vi "TDMS_CalcSize.vi"(7 "游标设定":T1={"初始Offset"=0, "每隔多少点读一次"=100000, "每次读的点数"=128}, 8 "错误输入":errorcluster, 9 "Cur2":cluster{"X":dbl, "Y":dbl}={"X"=31490.774276845874, "Y"=-0.08000000000000003}, 10 "Cur1":cluster{"X":dbl, "Y":dbl}={"X"=55721.10494959388, "Y"=0.43999999999999984}, 11 "tdms文件":refnum<k34>) -> (0 "错误输出":errorcluster, 1 "大于300M":bool, 2 "数据大小(MB)":dbl=1.7309100138019612e+18, 3 "tdms out":refnum<k34>)   [LabVIEW 2011]
panel:
  in  "通道名":string[](array[string])=["Sinc", "Sin"]
  in  "组名称输入":string="Sig Group"
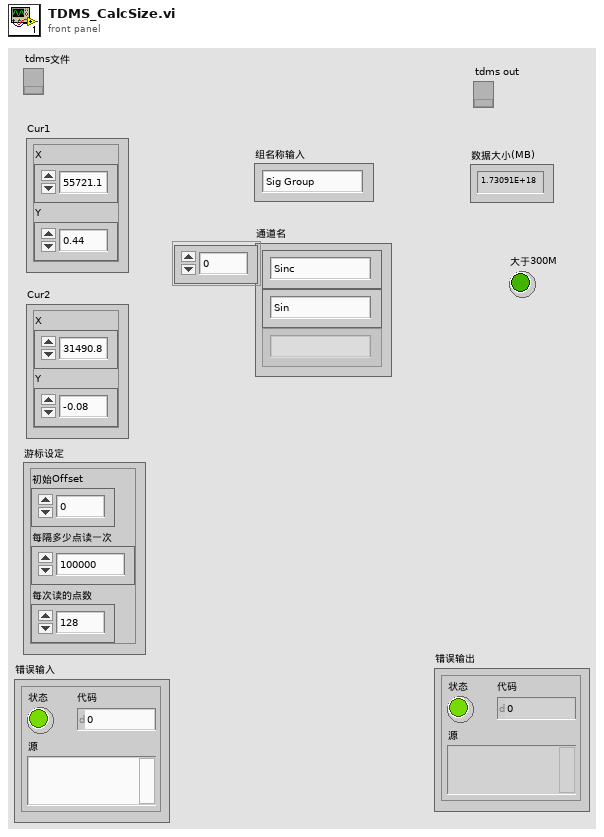
[diagram p1: front panel]
types:
  T1 = cluster{"初始Offset":u64, "每隔多少点读一次":u64, "每次读的点数":u64}
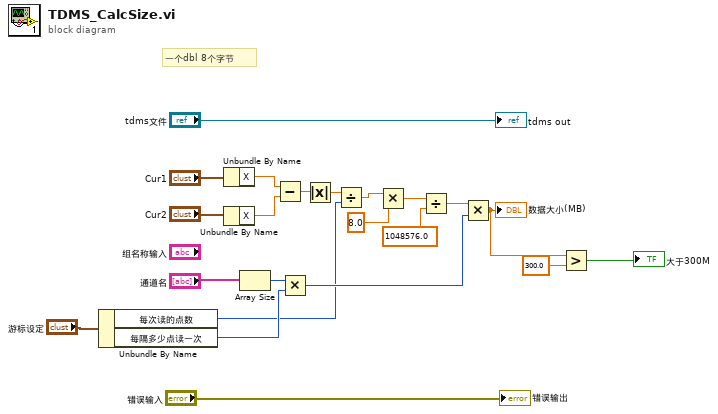
[diagram p0: block diagram]
diagram:
  # "一个dbl 8个字节"
  n1 = Unbundle By Name("游标设定") -> ("每次读的点数"=w4:u64, "每隔多少点读一次"=w7:u64)
  n2 = Unbundle By Name("Cur1") -> ("X"=w19:dbl)
  n3 = Unbundle By Name("Cur2") -> ("X"=w18:dbl)
  n4 = Array Size(array="通道名") -> (size(s)=w10:i32)
  n5 = Subtract(x=w19, y=w18) -> (x-y=w17:dbl)
  n6 = Multiply(x=w10, y=w7) -> (x*y=w9:u64)
  n7 = Absolute Value(x=w17) -> (abs(x)=w6:dbl)
  n8 = Divide(x=w6, y=w4) -> (x/y=w5:dbl)
  n9 = Multiply(x=w5, y=8.0) -> (x*y=w15:dbl)
  n10 = Divide(x=w15, y=1048576.0) -> (x/y=w12:dbl)
  n11 = Multiply(x=w12, y=w9) -> (x*y=w3:dbl)
  "数据大小(MB)" <- w3
  n12 = Greater?(x=w3, y=300.0) -> (0:→"大于300M":bool)
  "tdms out" <- "tdms文件"
  "错误输出" <- "错误输入"
